vi "Shutdown.vi"(11 "Sound Player in":refnum<class "Sound Player.lvclass">) -> (0 "error out":errorcluster, 3 "Sound Player out":refnum<class "Sound Player.lvclass">)   [LabVIEW 2017, in "Sound Player.lvclass"]
doc: "Do the work necessary to shut down the sound player. This includes closing references or windows or processes that were acquired/started by the sound player."
uses:
  Sound Player.lvclass
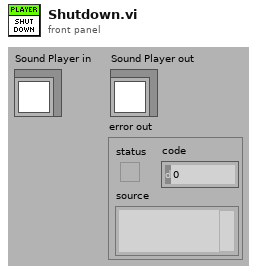
[diagram p1: front panel]
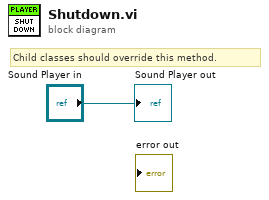
[diagram p0: block diagram]
diagram:
  # "Child classes should override this method."
  "Sound Player out" <- "Sound Player in"
